vi "_EnumEditor_CheckUnique.vi"(8 "error in (no error)":errorcluster, 11 "_EnumEditor in":refnum<class "_EnumEditor.lvclass">) -> (0 "error out":errorcluster, 3 "_EnumEditor out":refnum<class "_EnumEditor.lvclass">)   [LabVIEW 2014, in "_EnumEditor.lvclass"]
uses:
  _EnumEditor.lvclass
  _EnumEditor.lvclass/_EnumEditor.ctl
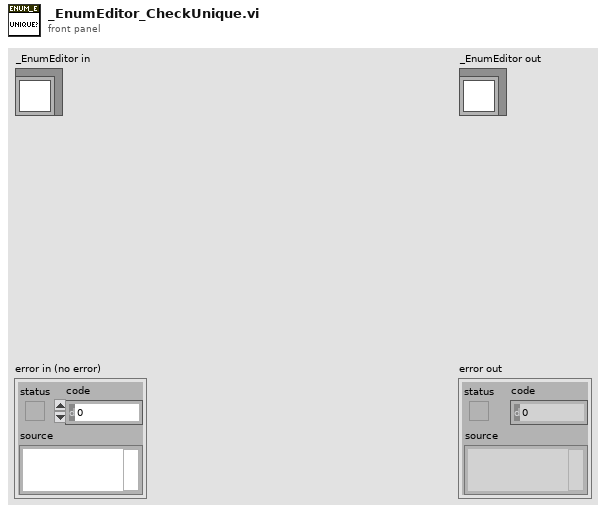
[diagram p1: front panel]
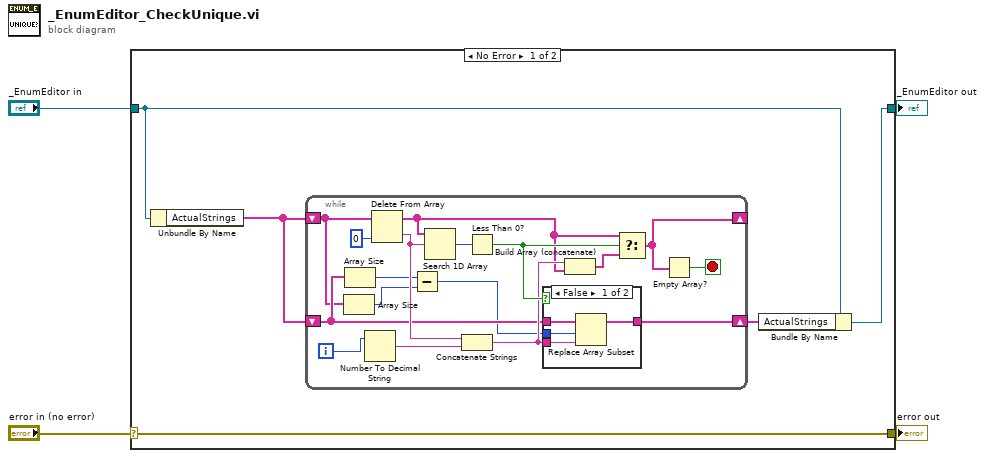
[diagram p0: block diagram]
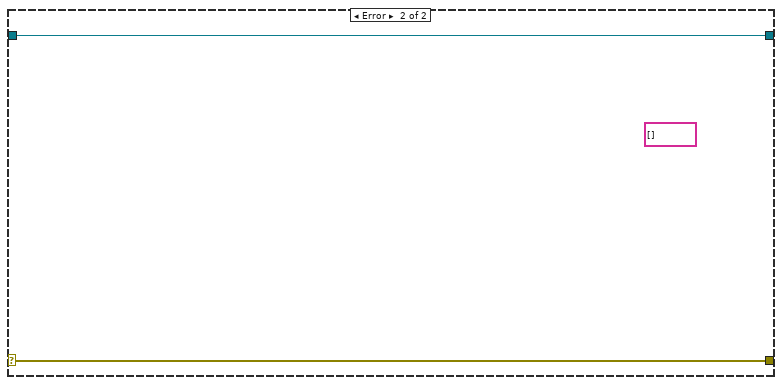
[diagram p3: hidden frame]
diagram:
  n1 = case shown="No Error" "error in (no error)" {
    selector: "error in (no error)" -> [w9 w33]
    tunnel: [w9 w33] -> w3
    tunnel: [w5 w32] -> w1
    tunnel: "_EnumEditor in" -> [w7 w32]
    frame No Error {
      n2 = Unbundle By Name(w7) -> ("ActualStrings"=w8:string[])
      n3 = while {
        shift-right: [w25] -> _
        shift-left: w8 -> [w13]
        shift-right: [w20] -> w6
        shift-left: w8 -> [w14]
        i -> [w16]
        stop <- w21 stop-if-true
        n4 = Array Size(array=w13) -> (size(s)=w11:i32)
        n5 = Array Size(array=w14) -> (size(s)=w12:i32)
        n6 = Number To Decimal String(number=w16) -> (decimal integer string=w22:string)  [unwired: 1 in]
        n7 = Delete From Array(array=w13, index=0) -> (deleted portion=w23:string, array with subset deleted=w15:string[])  [unwired: 1 in]
        n8 = Subtract(x=w12, y=w11) -> (x-y=w10:i32)
        n9 = Search 1D Array(1D array=w15, element=w23) -> (index of element=w24:i32)  [unwired: 1 in]
        n10 = Concatenate Strings(w23, w22) -> (w18:string)
        n11 = Less Than 0?(x=w24) -> (x < 0?=w19:bool)
        n12 = case shown="False" w19 {
          tunnel: w18 -> [w30 _]
          tunnel: w14 -> [w29 w31]
          tunnel: [w28 w31] -> w20
          tunnel: w10 -> [w27 _]
          frame False {
            n13 = Replace Array Subset(array=w29, new element=w30, index=w27) -> (w28:string[])
          }
          frame True {
          }
        }
        n14 = Build Array (concatenate)(w18, w15) -> (w17:string[])
        n15 = Select(t=w15, s=w19, f=w17) -> (s? t:f=w25:string[])
        n16 = Empty Array?(array=w25) -> (empty?=w21:bool)
      }
      n17 = Bundle By Name(cluster=w7, "ActualStrings"=w6) -> (w5:refnum<class "_EnumEditor.lvclass">)
    }
    frame Error {
      (unwired) string[] [] ("Array In")
    }
  }
  "error out" <- w3
  "_EnumEditor out" <- w1
